vi "Get Bmp Data.vi"(8 "错误输入":errorcluster, 9 "Offset":i32, 10 "Info Header In":T1, 11 "Bmp Data In":string) -> (0 "错误输出":errorcluster, 2 "Info Header Out":T1, 5 "Image Data":u8[](array[numeric]))   [LabVIEW 2012, in "Picture Box Tools.lvlib" / "BMP File.lvlib"]
uses:
  BMP File.lvlib
  Bmp Info Header.ctl
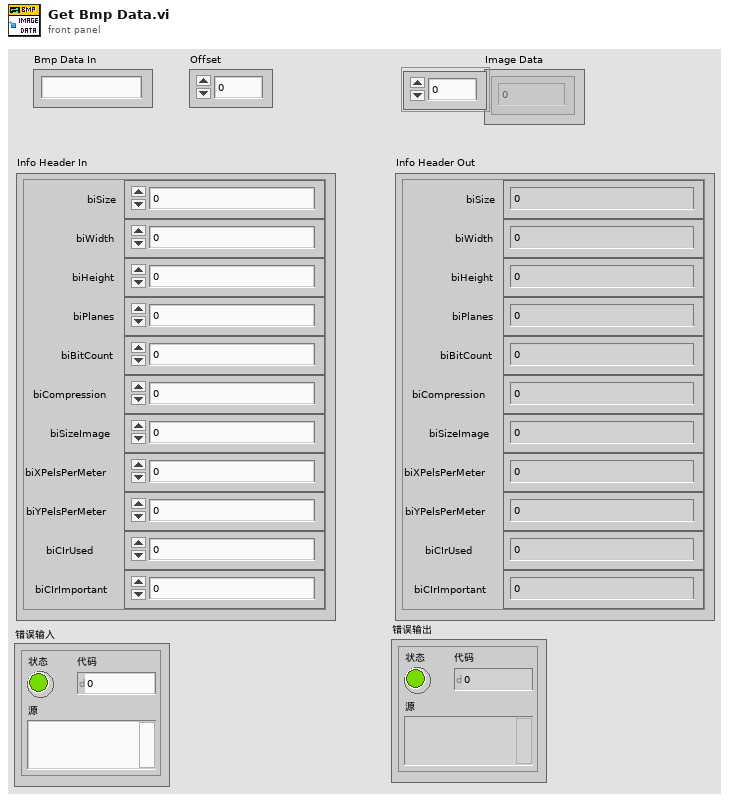
[diagram p1: front panel]
types:
  T1 = typedef "Picture Box Tools.lvlib/BMP File.lvlib/Bmp Info Header.ctl" = cluster{"biSize":u32, "biWidth":i32, "biHeight":i32, "biPlanes":u16, "biBitCount":u16, "biCompression":u32, "biSizeImage":u32, "biXPelsPerMeter":i32, "biYPelsPerMeter":i32, "biCIrUsed":u32, "biCIrImportant":u32}
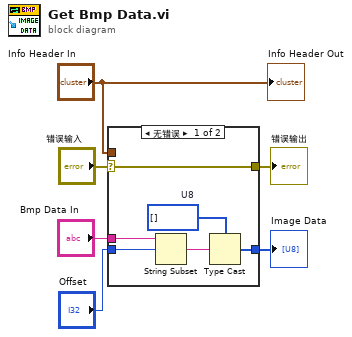
[diagram p0: block diagram]
diagram:
  n1 = case shown="无错误" "错误输入" {
    selector: "错误输入" -> [w7 w13]
    tunnel: "Info Header In" -> [_ _]
    tunnel: "Bmp Data In" -> [w11 _]
    tunnel: "Offset" -> [w12 _]
    tunnel: [w7 w13] -> w2
    tunnel: [w8 _] -> w1
    frame No Error {
      w9 = u8[] []  # U8
      n2 = String Subset(string=w11, offset (0)=w12) -> (substring=w10:string)  [unwired: 1 in]
      n3 = Type Cast(type=w9, x=w10) -> (*(type *) &x=w8:u8[])
    }
    frame Error {
    }
  }
  "错误输出" <- w2
  "Image Data" <- w1
  "Info Header Out" <- "Info Header In"
